vi "getSinglePointList.vi"(10 "XML document":path caption="XML文档路径", 11 "itemName":string) -> (3 "pointList":string[](array[string]))   [LabVIEW 2011]
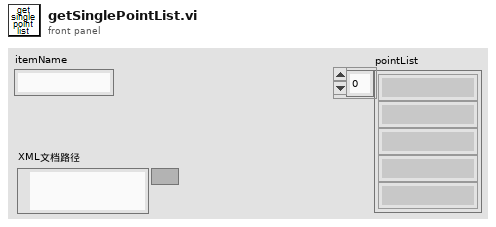
[diagram p1: front panel]
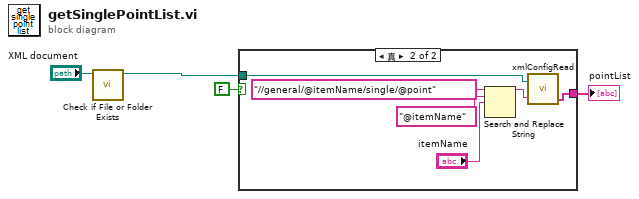
[diagram p0: block diagram]
diagram:
  n1 = call <vilib>:"Check if File or Folder Exists.vi"("path"="XML document") -> ("dup path"=w2:path)  [unwired: 8 in, 2 out]
  n2 = case shown="真" FALSE {
    tunnel: [_ w6] -> w3
    tunnel: w2 -> [_ w5]
    frame False {
    }
    frame True {
      n3 = Search and Replace String(input string="//general/@itemName/single/@point" ("XPath expression"), search string="@itemName" ("搜索字符串"), replace string="itemName") -> (result string=w10:string)  [unwired: 5 in, 3 out]
      n4 = call "xmlConfigRead.vi"("path to XML document"=w5, "XPath expression"=w10) -> ("OutParaArray"=w6:string[])  [unwired: 2 out]
    }
  }
  "pointList" <- w3
